vi "Drive convert linear feet and sensor units.vi"(2 "Drive position in (feet)":dbl, 3 "Drive position in (u)":dbl) -> (0 "Drive Position out (u)":dbl, 1 "Drive Position out (ft)":dbl)   [LabVIEW 2019]
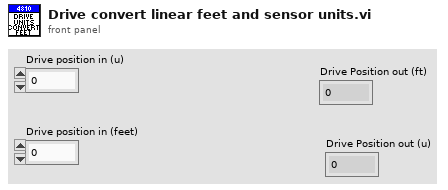
[diagram p1: front panel]
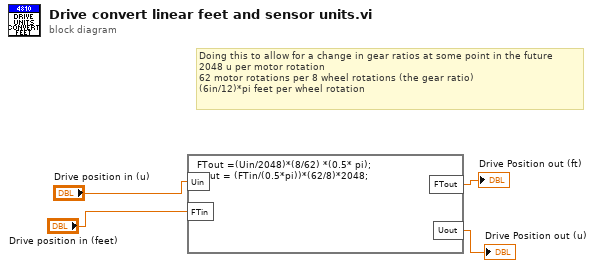
[diagram p0: block diagram]
diagram:
  # "Doing this to allow for a change in gear ratios at some point in the future\n2048 u per motor rotation\n62 motor rotations per 8 wheel rotations (the gear ratio)\n(6in/12)*pi feet per wheel rotation"
  n1 = formula code="FTout =(Uin/2048)*(8/62) *(0.5* pi);\nUout = (FTin/(0.5*pi))*(62/8)*2048;"("Uin"="Drive position in (u)", "FTin"="Drive position in (feet)") -> ("FTout"=→"Drive Position out (ft)":dbl, "Uout"=→"Drive Position out (u)":dbl)
